vi "Sensor ID.vi"(8 "error in (no error)":errorcluster, 11 "Scale in":refnum<class "Scale Config.lvclass">) -> (0 "error out":errorcluster, 2 "Sensor ID":string, 3 "Scale out":refnum<class "Scale Config.lvclass">)   [LabVIEW 2020, in "VolatusConfig.lvlib" / "Scale Config.lvclass"]
uses:
  Scale Config.lvclass
  C:/dev/lv20CE/relink/lv-volatus/VolatusConfig/VolatusConfigElement/VolatusConfigElement.lvclass
  VolatusConfigElement/VolatusConfigElement.lvclass/VolatusConfigElement.ctl
  VolatusConfigElement/Element.vi
  Scale Config.lvclass/Scale Config.ctl
  VolatusConfigElement/VolatusConfigElement.lvclass
  lv-cdm/CDM-Config/Config Element/Config Element.lvclass
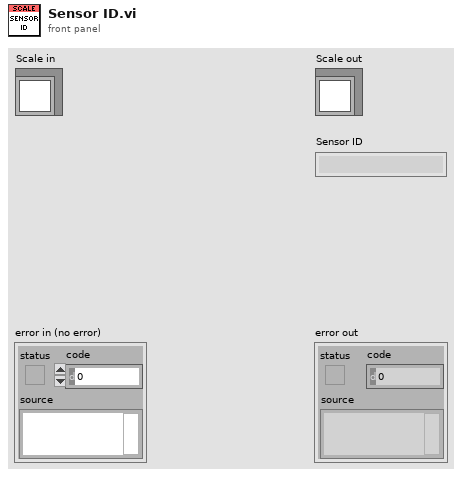
[diagram p1: front panel]
types:
  T1 = typedef "VolatusConfig.lvlib/Scale Type.ctl" = enum16{"None", "Sensor", "Polynomial", "Threshold", "Invert Bool", "Exponential"}
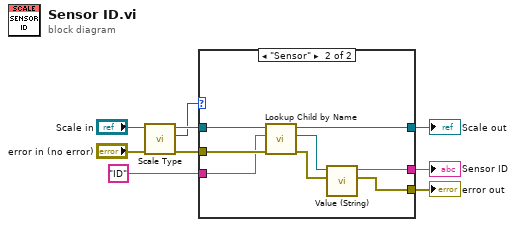
[diagram p0: block diagram]
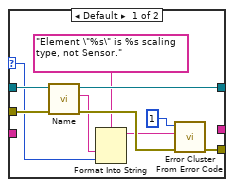
[diagram p2: hidden frame]
diagram:
  n1 = call "Scale Type.vi"("error in (no error)"="error in (no error)", "Scale in"="Scale in") -> ("error out"=w4:errorcluster, "Scale Type"=w1:T1, "Scale out"=w2:refnum<class "Scale Config.lvclass">)  [unwired: 7 in]
  n2 = case shown="\"Sensor\"" w1 {
    selector: w1 -> [w10 _]
    tunnel: [w15 w26] -> w8
    tunnel: "ID" ("Child Name") -> [_ w25]
    tunnel: [w17 w24] -> w6
    tunnel: [_ w23] -> w5
    tunnel: w4 -> [w14 w27]
    tunnel: w2 -> [w18 w22]
    frame Default {
      n3 = call "Name.vi"("error in (no error)"=w14, "VolatusConfigElement in"=w18) -> ("error out"=w19:errorcluster, "Name"=w13:string, "VolatusConfigElement out"=w15:refnum<class "Scale Config.lvclass">)  [unwired: 7 in]
      n4 = Format Into String(format string="Element \"%s\" is %s scaling type, not Sensor.", w13, w10) -> (resulting string=w12:string)  [unwired: 2 in, 1 out]
      n5 = call <vilib>:"Error Cluster From Error Code.vi"("error in (no error)"=w19, "error message (\"\")"=w12, "error code (0)"=1) -> ("error out"=w17:errorcluster)  [unwired: 6 in]
    }
    frame "Sensor" {
      n6 = call "Lookup Child by Name.vi"("error in (no error)"=w27, "Child Name"=w25, "VolatusConfigElement in"=w22) -> ("error out"=w20:errorcluster, "Child"=w21:refnum<class "Config Element.lvclass">, "VolatusConfigElement out"=w26:refnum<class "Scale Config.lvclass">)  [unwired: 5 in, 1 out]
      n7 = call "Value (String).vi"("error in (no error)"=w20, "Config Element in"=w21) -> ("error out"=w24:errorcluster, "String Value"=w23:string)  [unwired: 8 in]
    }
  }
  "error out" <- w6
  "Scale out" <- w8
  "Sensor ID" <- w5
